vi "Offset Widget Offset Values.vi"(7 "Force Offset Tag":string, 8 "Coordinate Space":bool caption="Coord", 9 "Rigid Connection In":bool, 10 "Number of\nLBCBs":T1, 11 "Offset Type":T2) -> (3 "Offsets":dbl[][](array[numeric]))   [LabVIEW 2013]
uses:
  Apps/Yes No Button.ctl
  Global Data/Transactions/Dataset Type.ctl
  Global Data/Transactions/Dataset Source.ctl
  Global Data/Transactions/Dataset Transaction Id.ctl
  Offsets/Offset Types.ctl
  Data Access Objects/Application/Number Of LBCBs.ctl
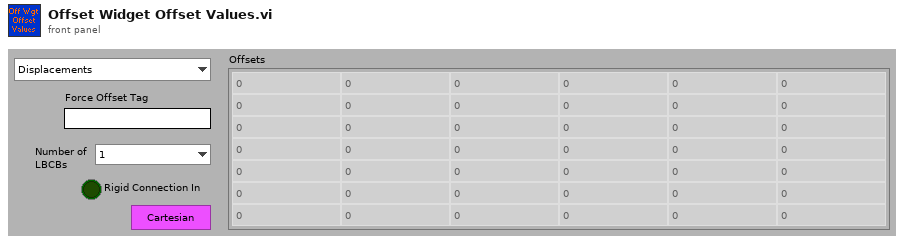
[diagram p1: front panel]
types:
  T1 = typedef "Number Of LBCBs.ctl" = enum16{"1", "2"}
  T2 = typedef "Offset Types.ctl" = enum16{"Displacements", "Forces", "External Sensors"}
  T3 = typedef "Dataset Transaction Id.ctl" = cluster{"Dataset Source":T4, "Dataset Type":T5, "Hold":T6, "Volts":T6, "Tag":string}
  T4 = typedef "Dataset Source.ctl" = enum16{"Continuous", "Hold", "ED", "Volts", "Offsets", "Increments"}
  T5 = typedef "Dataset Type.ctl" = enum16{"LVDT", "Load Cell", "Actuator Command", "Servo Error", "Displacement Command", "Displacement", "Force"}
  T6 = typedef "Yes No Button.ctl" = bool
  T7 = typedef "Dataset Source.ctl" = enum16{"LBCB 1", "LBCB 2", "Combined", "External Sensors"}
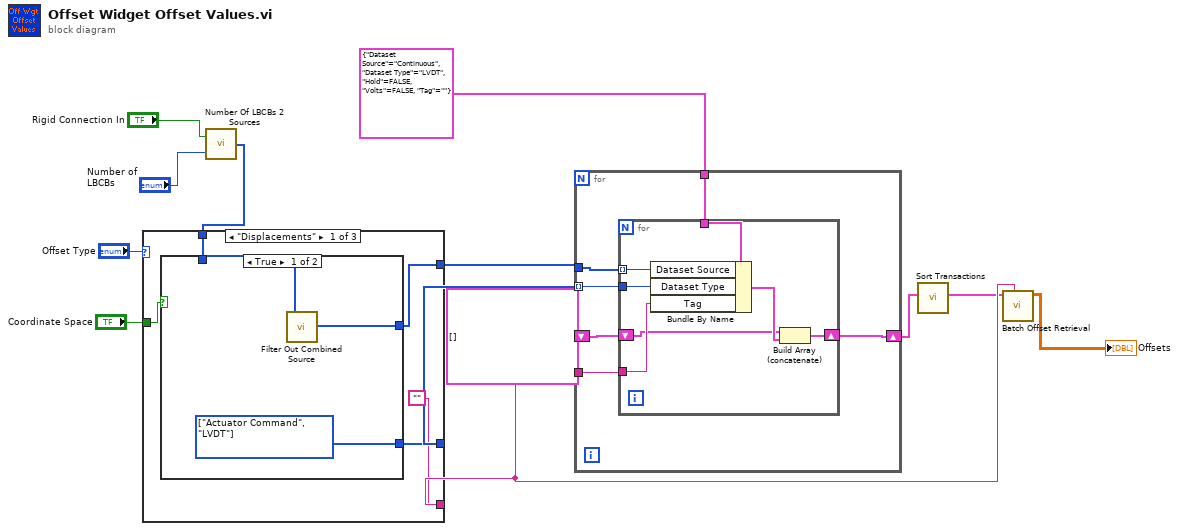
[diagram p0: block diagram]
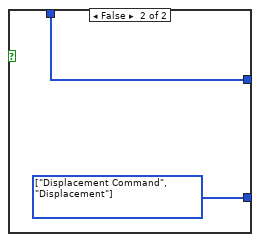
[diagram p2: hidden frame]
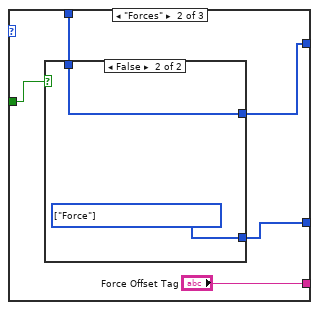
[diagram p3: hidden frame]
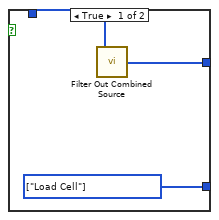
[diagram p4: hidden frame]
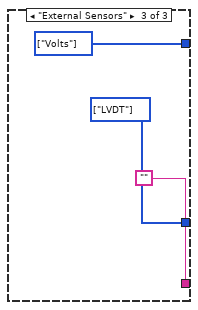
[diagram p5: hidden frame]
diagram:
  n1 = call "Number Of LBCBs 2 Sources.vi"("Number of LBCBs"="Number of\nLBCBs", "Combined LBCBs"="Rigid Connection In") -> ("Sources"=w3:T7[])
  n2 = case shown="\"Displacements\"" "Offset Type" {
    tunnel: "Coordinate Space" -> [w18 w28 _]
    tunnel: [w17 w27 w36] -> w8
    tunnel: ["" "Force Offset Tag" ""] -> w5
    tunnel: w3 -> [w15 w25 _]
    tunnel: [w14 w24 w34] -> w2
    frame "Displacements" {
      n3 = case shown="True" w18 {
        tunnel: [w21 w23] -> w17
        tunnel: w15 -> [w20 w22]
        tunnel: [w19 w22] -> w14
        frame True {
          w21 = T5[] [enum."Actuator Command", enum."LVDT"] items=["LVDT", "Load Cell", "Actuator Command", "Servo Error", "Displacement Command", "Displacement", "Force"]
          n4 = call "Filter Out Combined Source.vi"("Sources In"=w20) -> ("Sources Out"=w19:T4[])
        }
        frame False {
          w23 = T5[] [enum."Displacement Command", enum."Displacement"] items=["LVDT", "Load Cell", "Actuator Command", "Servo Error", "Displacement Command", "Displacement", "Force"]
        }
      }
    }
    frame "Forces" {
      n5 = case shown="False" w28 {
        tunnel: [w31 w33] -> w27
        tunnel: w25 -> [w30 w32]
        tunnel: [w29 w32] -> w24
        frame True {
          w31 = T5[] [enum."Load Cell"] items=["LVDT", "Load Cell", "Actuator Command", "Servo Error", "Displacement Command", "Displacement", "Force"]
          n6 = call "Filter Out Combined Source.vi"("Sources In"=w30) -> ("Sources Out"=w29:T4[])
        }
        frame False {
          w33 = T5[] [enum."Force"] items=["LVDT", "Load Cell", "Actuator Command", "Servo Error", "Displacement Command", "Displacement", "Force"]
        }
      }
    }
    frame "External Sensors" {
      w34 = T4[] [enum."Volts"] items=["Continuous", "Hold", "ED", "Volts", "Offsets", "Increments"] ("Sources")
      w36 = T5[] [enum."LVDT"] items=["LVDT", "Load Cell", "Actuator Command", "Servo Error", "Displacement Command", "Displacement", "Force"]
    }
  }
  n7 = for {
    tunnel: w2 -> [w40]
    tunnel: T3 {"Dataset Source"=enum."Continuous", "Dataset Type"=enum."LVDT", "Hold"=FALSE, "Volts"=FALSE, "Tag"=""} ("Dataset Trans Id") -> [w42]
    tunnel: w5 -> [w41]
    tunnel: w8 -> [w39] mode=indexing
    shift-right: [w38] -> w7
    shift-left: T3[] [] -> [w37]
    n8 = for {
      tunnel: w42 -> [w49]
      tunnel: w41 -> [w48]
      tunnel: w40 -> [w47] mode=indexing
      tunnel: w39 -> [w46]
      shift-right: [w44] -> w38
      shift-left: w37 -> [w43]
      n9 = Bundle By Name(cluster=w49, "Dataset Source"=w47, "Dataset Type"=w46, "Tag"=w48) -> (w45:T3)
      n10 = Build Array (concatenate)(w43, w45) -> (w44:T3[])
    }
  }
  n11 = call "Sort Transactions.vi"("Transactions In"=w7) -> ("Transactions Out"=w1:T3[])  [unwired: 10 in]
  n12 = call "Batch Offset Retrieval.vi"("Tag"=w5, "Transactions"=w1) -> ("Data"=→"Offsets":dbl[][])  [unwired: 8 in, 1 out]
